vi "TSC.vi"(0 "参数":string[](array[string])=["123456789123456", "", "", "10000", "", "", "21214", "", "512", "PASS"]) -> ()   [LabVIEW 2020]
uses:
  <vilib>/Utility/NIReport.llb/Report Type.ctl
  <vilib>/Utility/NIReport.llb/NI_report.lvclass
  <vilib>/Utility/NIReport.llb/NI_ReportGenerationCore.lvlib
  <vilib>/Utility/NIReport.llb/Excel/NI_Excel.lvclass
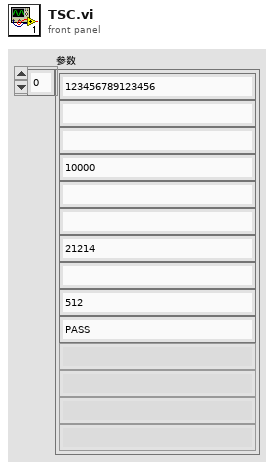
[diagram p1: front panel]
types:
  T1 = typedef "NI_ReportGenerationCore.lvlib/Report Type.ctl" = enum16{"HTML", "Word", "Excel"}
  T2 = enum16{"maximized", "minimized", "normal", "no change"}
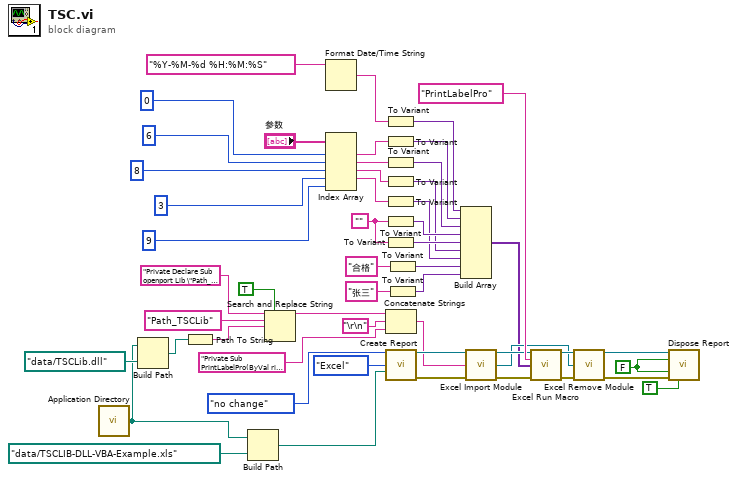
[diagram p0: block diagram]
diagram:
  w19 = ""
  w34 = FALSE ("wait until printing completed? (T)")
  n1 = call <vilib>:"Application Directory.vi"() -> ("Application Directory"=w31:path)
  n2 = Build Path(base path=w31, name or relative path=path "data/TSCLib.dll") -> (appended path=w35:path)
  n3 = Path To String(path=w35) -> (string=w38:string)
  n4 = Build Path(base path=w31, name or relative path=path "data/TSCLIB-DLL-VBA-Example.xls" ("template (empty)")) -> (appended path=w32:path)
  n5 = Search and Replace String(replace all?=TRUE ("replace all? (F)"), input string="Private Declare Sub openport Lib \"Path_TSCLib\" (ByVal PrinterName As String)\nPrivate Declare Sub closeport Lib \"Path_TSCLib\" ()\nPrivate Declare Sub sendcommand Lib \"Path_TSCLib\" (ByVal command As String)\nPrivate Declare Sub setup Lib \"Path_TSCLib\" ( _\n        ByVal LabelWidth As String, _\n        ByVal LabelHeight As String, _\n        ByVal Speed As String, _\n        ByVal Density As String, _\n        ByVal Sensor As String, _\n        ByVal Vertical As String, _\n        ByVal Offset As String)\nPrivate Declare Sub downloadpcx Lib \"Path_TSCLib\" ( _\n        ByVal Filename As String, _\n        ByVal ImageName As String)\nPrivate Declare Sub barcode Lib \"Path_TSCLib\" ( _\n        ByVal X As String, _\n    ByVal Y As String, _\n    ByVal CodeType As String, _\n    ByVal Height As String, _\n    ByVal Readable As String, _\n    ByVal rotation As String, _\n    ByVal Narrow As String, _\n    ByVal Wide As String, _\n    ByVal Code As String)\nPrivate Declare Sub printerfont Lib \"Path_TSCLib\" ( _\n    ByVal X As String, _\n    ByVal Y As String, _\n    ByVal FontName As String, _\n    ByVal rotation As String, _\n    ByVal Xmul As String, _\n    ByVal Ymul As String, _\n    ByVal Content As String)\nPrivate Declare Sub clearbuffer Lib \"Path_TSCLib\" ()\nPrivate Declare Sub printlabel Lib \"Path_TSCLib\" ( _\n    ByVal NumberOfSet As String, _\n    ByVal NumberOfCopy As String)\nPrivate Declare Sub formfeed Lib \"Path_TSCLib\" ()\nPrivate Declare Sub nobackfeed Lib \"Path_TSCLib\" ()\nPrivate Declare Sub windowsfont Lib \"Path_TSCLib\" ( _\n    ByVal X As Integer, _\n    ByVal Y As Integer, _\n    ByVal fontheight As Integer, _\n    ByVal rotation As Integer, _\n    ByVal fontstyle As Integer, _\n    ByVal fontunderline As Integer, _\n    ByVal FaceName As String, _\n    ByVal TextContent As String)\n\nPrivate Declare Sub windowsfontU Lib \"Path_TSCLib\" ( _\n    ByVal X As Integer, _\n    ByVal Y As Integer, _\n    ByVal fontheight As Integer, _\n    ByVal rotation As Integer, _\n    ByVal fontstyle As Integer, _\n    ByVal fontunderline As Integer, _\n    ByVal FaceName As String, _\n    ByVal TextContent As String)\n\nPrivate Declare Sub about Lib \"Path_TSCLib\" ()\n\nPrivate Declare Function isusbportready Lib \"Path_TSCLib\" () As Integer\nPrivate Declare Function usbportqueryprinter Lib \"Path_TSCLib\" () As Integer\nPrivate Declare Function usbportwrite Lib \"Path_TSCLib\" (ByVal command As String) As Integer\n\n" ("module code (\"\")"), search string="Path_TSCLib", replace string=w38) -> (result string=w1:string)  [unwired: 4 in, 3 out]
  n6 = Format Date/Time String(time format string (%c)="%Y-%M-%d %H:%M:%S") -> (date/time string=w22:string)  [unwired: 2 in]
  n7 = Index Array(array="参数", index #1=0 ("index"), index #2=6 ("index"), index #3=8 ("index"), index #4=3 ("index"), index #5=9 ("index")) -> (element #1=w21:string, element #2=w20:string, element #3=w18:string, element #4=w17:string)  [unwired: 1 out]
  n8 = To Variant(anything=w22) -> (Variant=w14:variant)
  n9 = To Variant(anything=w21) -> (Variant=w13:variant)
  n10 = To Variant(anything=w20) -> (Variant=w12:variant)
  n11 = To Variant(anything=w18) -> (Variant=w6:variant)
  n12 = To Variant(anything=w17) -> (Variant=w9:variant)
  n13 = To Variant(anything=w19) -> (Variant=w11:variant)
  n14 = To Variant(anything=w19) -> (Variant=w10:variant)
  n15 = Concatenate Strings(w1, "\r\n", "Private Sub PrintLabelPro(ByVal riqi As String, cpxh As String, jcyl As String, cqsj As String, phsj As String, cssj As String, xll As String, csjg As String, jyy As String)\n    Call openport(\"TSC DC2700\")\n    Call setup(\"101.6\", \"39.54\", \"5\", \"11\", \"0\", \"3\", \"0\")\n    Call clearbuffer\n    Call sendcommand(\"DIRECTION 1\")\n    Call windowsfont(205, 10, 30, 0, 0, 0, \"宋体\", [B1].Value)\n    Call windowsfont(135, 60, 30, 0, 0, 0, \"宋体\", [A2].Value + riqi)\n    Call windowsfont(135, 100, 30, 0, 0, 0, \"宋体\", [A3].Value + cpxh + \"  \" + [C3].Value + jcyl)\n    Call windowsfont(135, 140, 30, 0, 0, 0, \"宋体\", [A4].Value + [B4].Value + \"  \" + [C4].Value + [D4].Value)\n    Call windowsfont(135, 180, 30, 0, 0, 0, \"宋体\", [A5].Value + [B5].Value + \"  \" + [C5].Value + xll)\n    Call windowsfont(135, 220, 30, 0, 0, 0, \"宋体\", [A6].Value + csjg + \"  \" + [C6].Value + [D6].Value)\n'    Call windowsfont(135, 260, 30, 0, 0, 0, \"宋体\", [A7].Value + \"\" + [B7].Value + \"   \" + [C7].Value + \"\" + [D7].Value)\n    Call sendcommand(\"SET CUTTER 1\")\n    Call printlabel(\"1\", \"1\")\n    Call closeport\nEnd Sub" ("module code (\"\")")) -> (w4:string)
  n16 = call <vilib>:"Create Report.vi"("window state (normal)"=T2."no change", "report type"=Report_Type."Excel", "template (empty)"=w32) -> ("report out"=w47:refnum<class "NI_report.lvclass">, "error out"=w48:errorcluster)  [unwired: 11 in]
  n17 = To Variant(anything="合格" ("time format string (%c)")) -> (Variant=w8:variant)
  n18 = To Variant(anything="张三" ("time format string (%c)")) -> (Variant=w7:variant)
  n19 = Build Array(w14, w13, w12, w11, w10, w6, w9, w8, w7) -> (w5:variant[])
  n20 = call <vilib>:"Excel Import Module.vi"("report in"=w47, "module code (\"\")"=w4, "error in (no error)"=w48) -> ("report out"=w46:refnum<class "NI_report.lvclass">, "module reference"=w37:refnum<k7>, "error out"=w45:errorcluster)  [unwired: 10 in]
  n21 = call <vilib>:"Excel Run Macro.vi"("report in"=w46, "macro name"="PrintLabelPro", "parameters"=w5, "error in (no error)"=w45) -> ("report out"=w44:refnum<class "NI_report.lvclass">, "error out"=w43:errorcluster)  [unwired: 9 in, 1 out]
  n22 = call <vilib>:"Excel Remove Module.vi"("report in"=w44, "module reference"=w37, "error in (no error)"=w43) -> ("report out"=w42:refnum<class "NI_report.lvclass">, "error out"=w41:errorcluster)  [unwired: 11 in]
  n23 = call-dynamic "Dispose Report.vi"("report in"=w42, "wait until printing completed? (T)"=w34, "save changes? (F)"=w34, "error in (no error)"=w41, "close report? (T)"=TRUE ("wait until printing completed? (T)")) -> ()  [unwired: 10 in, 1 out]
